vi "XIPIN_3GPP_Downlink_Chip_Rate_1_0.vi"   [LabVIEW 2017]
doc: "The 3GPP Downlink Chip Rate core provides a Release 6 Compliant, Xilinx FPGA optimized solution for Femto-cell, Pico-cell and Macro-cell solutions.The Xilinx Downlink Chip Rate LogiCORE is fully synchronous, using a single clock. The Downlink Chip Rate Core incorporates Xilinx Smart-IP technology for maximum performance. The core is delivered through the Xilinx CORE Generator System and integrates seamlessly with the Xilinx design flow.\n------------------------------------\n<b>Need License</b> : Yes"
uses:
  <vilib>/rvi/XilinxIP/XIPIN_XNode/niFpgaXIPIN.xnode
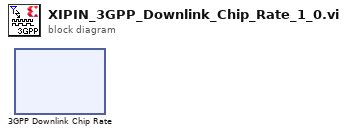
[diagram p0: block diagram]
diagram:
  n1 = xnode ("3GPP Downlink Chip Rate")() -> ()
